vi "rqcBob Configure SPD Detection Window (2PD).vi"(8 "error in":errorcluster, 9 "PD2.detection window":u8, 10 "PD1.detection window":u8, 11 "FPGA reference in":refnum<k20>) -> (0 "error out":errorcluster, 3 "FPGA reference out":refnum<k20>)   [LabVIEW 2019]
uses:
  <vilib>/Utility/error.llb/Error Cluster From Error Code.vi
  <vilib>/rvi/errors/niLvFpgaAdjustHostInterfaceError.vi
  <vilib>/rvi/interface/nirviReadWriteControl/nirviReadWriteControl.xnode
  NiFpgaLv.dll
  <vilib>/rvi/interface/Simulation/niFpgaSimulationCallBeginRW.vi
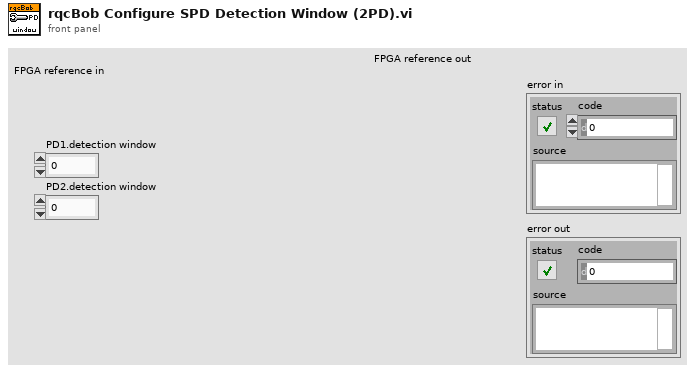
[diagram p1: front panel]
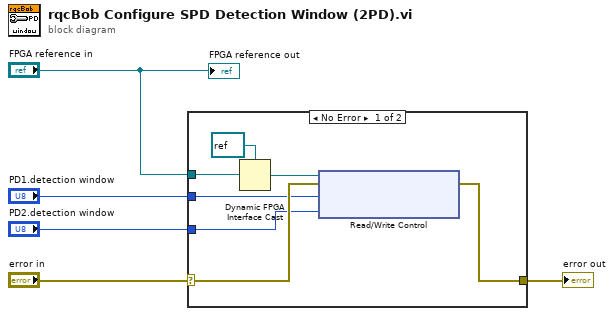
[diagram p0: block diagram]
diagram:
  n1 = case shown="No Error" "error in" {
    selector: "error in" -> [w12 w13]
    tunnel: [w11 w13] -> w3
    tunnel: "FPGA reference in" -> [w10 _]
    tunnel: "PD1.detection window" -> [w8 _]
    tunnel: "PD2.detection window" -> [w7 _]
    frame No Error {
      n2 = Dynamic FPGA Interface Cast(Session In=refnum<k20> refnum ("FPGA Interface"), Type=w10) -> (Session Out=w9:refnum<k20>)
      n3 = xnode "Read/Write Control"("FPGA VI Reference In"=w9, "error in"=w12, "PD1.detection window"=w8, "PD2.detection window"=w7) -> ("error out"=w11:errorcluster)  [unwired: 1 out]
    }
    frame Error {
    }
  }
  "error out" <- w3
  "FPGA reference out" <- "FPGA reference in"
